vi "Timeout.vi"(8 "Start Time In":u32, 11 "Time Limit":u32) -> (0 "Start Time Out":u32, 3 "Timeout":bool)   [LabVIEW 2016]
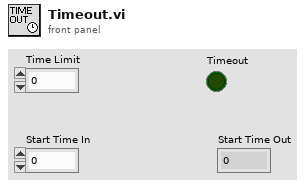
[diagram p1: front panel]
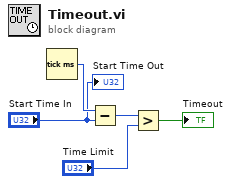
[diagram p0: block diagram]
diagram:
  n1 = Tick Count (ms)() -> (millisecond timer value=w5:u32)
  n2 = Subtract(x=w5, y="Start Time In") -> (x-y=w4:u32)
  n3 = Greater?(x=w4, y="Time Limit") -> (0:→"Timeout":bool)
  "Start Time Out" <- "Start Time In"
